vi "TDM Transmit Receive Test.vi"(6 "ready for output":bool, 7 "transfer":bool, 9 "input valid":bool, 10 "transfer length":u8=32, 11 "sample in":u32) -> (1 "output valid":bool, 2 "signals out":cluster{"clock":bool, "sync":bool, "sdata":bool}, 3 "sample out":u32, 4 "ready for input":bool)   [LabVIEW 2013]
uses:
  <vilib>/Platform/TimedLoop/XDataNode/timing_clust.ctl
  <vilib>/Platform/TimedLoop/XDataNode/nitl_modes.ctl
  <vilib>/Platform/TimedLoop/XDataNode/wakeup.ctl
  Source/Controls/tdm configuration.ctl
  <vilib>/rvi/Emulation/niFpgaSctlEmulationGetInTimedLoop.vi
  <vilib>/rvi/Emulation/niFpgaEmulationReportErrorSimple.vi
  <vilib>/rvi/Emulation/niFpgaGetClockAttributes.vi
  <vilib>/rvi/Emulation/niFpgaCriticalErrorInLSC.vi
  <vilib>/Platform/TimedLoop/XDataNode/XDataNode.xnode
  <vilib>/Platform/TimedLoop/XDataNode/XDNodeRunTimeDep.lvlib
  Source/I2S-TDM.lvlib
panel:
  in  "channel count":u8=2
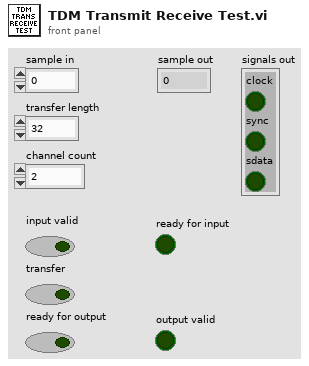
[diagram p1: front panel]
types:
  T1 = typedef "XDNodeRunTimeDep.lvlib/timing_clust.ctl" = cluster{"Expected End [f-1]":u64, "Actual End [f-1]":u64, "Finished Late? [f-1]":bool, "Expected End [i-1]":u64, "Actual End [i-1]":u64, "Finished Late? [i-1]":bool, "Expected Start [i]":u64, "Actual Start [i]":u64, "Expected Start [f]":u64, "Actual Start [f]":u64, "Source Name":string, "Structure Name":string, "Period":i64, "Deadline":i64, "Offset":i64, "Start":i64, "Priority":i32, "Timeout":i32, "Mode":T2, "Wakeup Reason":T3, "Error":errorcluster, "Source Type":string, "Secondary Source Type":string, "Global End Time":u64, "Global Start Time":u64, "Frame Duration":u64, "Iteration Duration":u64, "Assigned CPU":i32, "I/O Scan Engine Mode":u32}
  T2 = typedef "XDNodeRunTimeDep.lvlib/nitl_modes.ctl" = enum32{"No Change", "Process missed periods, maintain original phase", "Discard missed periods, maintain original phase", "Process missed periods, ignore original phase", "Discard missed periods, ignore original phase"}
  T3 = typedef "XDNodeRunTimeDep.lvlib/wakeup.ctl" = enum32{"Normal", "Aborted", "Asynchronous wakeup", "Timing source error", "Timed loop error", "Timeout"}
  T4 = enum16{"Sample Clock", "Pre-Start Pulse", "Word Select (I2S only)"}
  T5 = cluster{"Number of Channels":u8, "Bits Per Channel":u8, "Data Sample Edge":enum16{"rising", "falling"}, "Sync Format":enum16{"Sample Clock", "Pre-Start Pulse", "Word Select (I2S only)"}, "Inverted Sync":bool}
  T6 = typedef "I2S-TDM.lvlib/tdm configuration.ctl" = cluster{"Number of Channels":u8, "Bits Per Channel":u8, "Bit Set Edge":enum16{"rising", "falling"}, "Invert Frame Sync":bool}
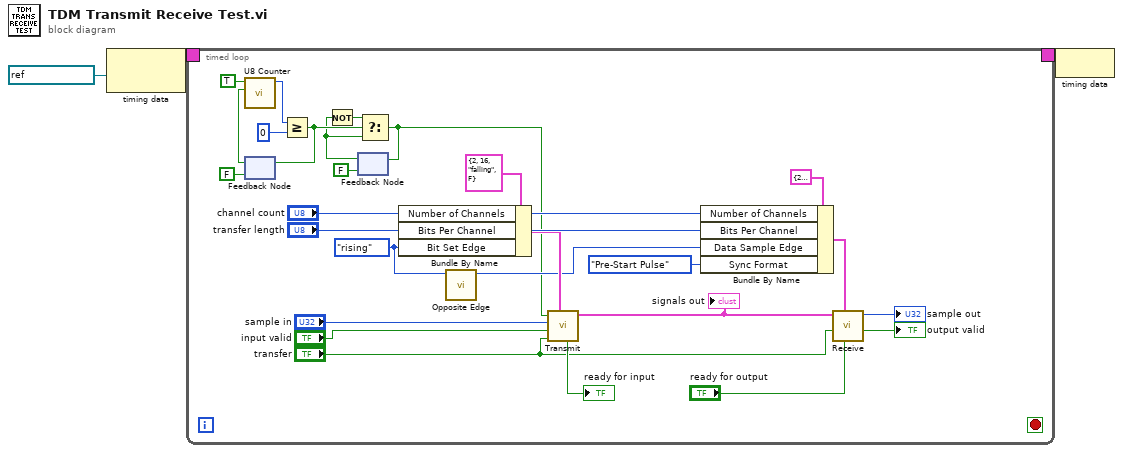
[diagram p0: block diagram]
diagram:
  n1 = node-c288(refnum<k21> "24.576MHz" ("Source Name")) -> (w3:T1)
  n2 = timed-loop {
    timing: w3 -> [_]
    timing-out: [_] -> w2
    stop <- _ stop-if-true
    w16 = enum16{"rising", "falling"}."rising" ("Bit Set Edge")
    n3 = feedback #1(FALSE) -> (w7:bool)
    n4 = call "U8 Counter.vi"("reset (F)"=w7, "increment"=TRUE) -> ("count"=w9:u8)  [unwired: 9 in]
    n5 = Greater Or Equal?(x=w9, y=u8 0) -> (x >= y?=w12:bool)
    n6 = feedback-in #1(w12) -> ()
    n7 = feedback #2(FALSE) -> (w11:bool)
    n8 = Not(x=w11) -> (.not. x?=w5:bool)
    n9 = Select(t=w5, s=w12, f=w11) -> (s? t:f=w4:bool)
    n10 = feedback-in #2(w4) -> ()
    n11 = Bundle By Name(cluster=T6 {"Number of Channels"=2, "Bits Per Channel"=16, "Bit Set Edge"=enum."falling", "Invert Frame Sync"=FALSE} ("Configuration"), "Number of Channels"="channel count", "Bits Per Channel"="transfer length", "Bit Set Edge"=w16) -> (w17:T6)
    n12 = call "Opposite Edge.vi"("edge in"=w16) -> ("opposite edge out"=w15:enum16{"rising", "falling"})  [unwired: 10 in]
    n13 = call "Transmit.vi"("configuration"=w17, "transmit"="transfer", "input valid"="input valid", "sample"="sample in", "clock in"=w4) -> ("signals out"=w26:cluster{"clock":bool, "sync":bool, "sdata":bool}, "ready for input"=→"ready for input":bool)  [unwired: 5 in]
    "signals out" <- w26
    n14 = Bundle By Name(cluster=T5 {"Number of Channels"=2, "Bits Per Channel"=16, "Data Sample Edge"=enum."falling", "Sync Format"=enum."Sample Clock", "Inverted Sync"=FALSE} ("configuration"), "Number of Channels"="channel count", "Bits Per Channel"="transfer length", "Data Sample Edge"=w15, "Sync Format"=T4."Pre-Start Pulse") -> (w20:T5)
    n15 = call "Receive.vi"("ready for output"="ready for output", "configuration"=w20, "receive"="transfer", "signals in"=w26) -> ("output valid"=→"output valid":bool, "sample"=→"sample out":u32)  [unwired: 6 in]
  }
  n16 = node-c288(w2) -> ()
